vi "Apply Pitch Bend.vi"(9 "Pitch Bend Up (F)":bool, 10 "Pitch Bend Down (F)":bool, 11 "Pitch (decimal) In":dbl) -> (3 "Pitch (decimal) Out":dbl)   [LabVIEW 2019, in "Audio Processing.lvlib"]
doc: "Apply pitch bend value to pitch decimal value (add or subtract 0.08, or 8%)."
uses:
  Audio Processing.lvlib
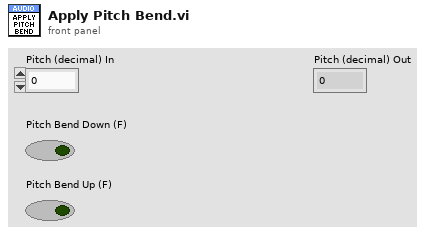
[diagram p1: front panel]
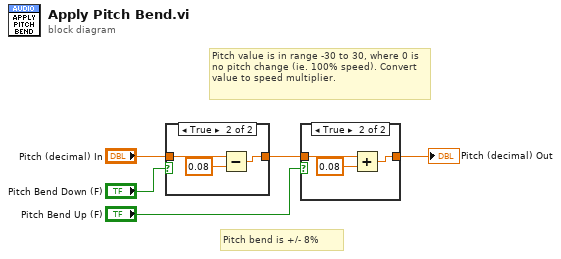
[diagram p0: block diagram]
diagram:
  # "Pitch bend is +/- 8%"
  # "Pitch value is in range -30 to 30, where 0 is no pitch change (ie. 100% speed). Convert value to speed multiplier."
  n1 = case shown="True" "Pitch Bend Down (F)" {
    tunnel: "Pitch (decimal) In" -> [w6 w9]
    tunnel: [w6 w7] -> w5
    frame False {
    }
    frame True {
      n2 = Subtract(x=w9, y=0.08) -> (x-y=w7:dbl)
    }
  }
  n3 = case shown="True" "Pitch Bend Up (F)" {
    tunnel: w5 -> [w10 w13]
    tunnel: [w10 w11] -> w1
    frame False {
    }
    frame True {
      n4 = Add(x=w13, y=0.08) -> (x+y=w11:dbl)
    }
  }
  "Pitch (decimal) Out" <- w1
